vi "PromVIEW_GlobalInit.vi"(11 "Item Ref":T1) -> ()   [LabVIEW 2020]
uses:
  <resource>/Framework/Providers/API/ItemRef.ctl
  <resource>/Framework/Providers/API/mxLvMenuItem.ctl
panel:
  out "error out":errorcluster
  in  "error in":errorcluster
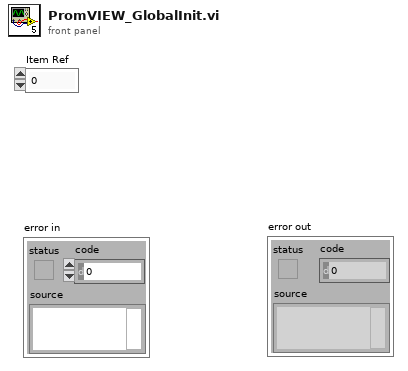
[diagram p1: front panel]
types:
  T1 = typedef "ItemRef.ctl" = u64
  T2 = enum32{"<None>", "Project", "Project / Build Specifications", "Tools", "Tools / Source Control", "Tools / Real-Time Module", "Help"}
  T3 = typedef "mxLvMenuItem.ctl" = cluster{"Menu Name":string, "Description":string, "Icon File Name":path, "Menu Tag":string, "Enabled":bool, "Checked":bool, "Separator":bool, "Batchable":bool, "Weight":i32, "Batch Mode (Ignored if Not Batchable)":enum32{"Show If All Items Support Command", "Show If Any Items Support Command"}, "Menu Location":enum32{"<None>", "Project", "Project / Build Specifications", "Tools", "Tools / Source Control", "Tools / Real-Time Module", "Help"}, "Exclude From Getting Started Window Menu":bool}
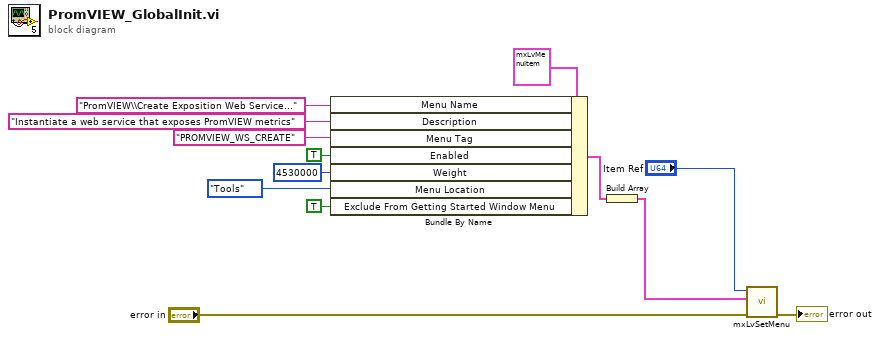
[diagram p0: block diagram]
diagram:
  n1 = Bundle By Name(cluster=T3 {"Menu Name"="", "Description"="", "Icon File Name"=path "", "Menu Tag"="", "Enabled"=TRUE, "Checked"=FALSE, "Separator"=FALSE, "Batchable"=TRUE, "Weight"=0, "Batch Mode (Ignored if Not Batchable)"=enum."Show If All Items Support Command", "Menu Location"=enum."<None>", "Exclude From Getting Started Window Menu"=FALSE} ("Menu Item"), "Menu Name"="PromVIEW\\Create Exposition Web Service...", "Description"="Instantiate a web service that exposes PromVIEW metrics", "Menu Tag"="PROMVIEW_WS_CREATE", "Enabled"=TRUE, "Weight"=4530000, "Menu Location"=T2."Tools", "Exclude From Getting Started Window Menu"=TRUE) -> (w9:T3)
  n2 = Build Array(w9) -> (w1:T3[])
  n3 = call <resource>:"mxLvSetMenu.vi"("error in"="error in", "Menu Items"=w1, "Item"="Item Ref") -> ("error out"=→"error out":errorcluster)  [unwired: 7 in, 1 out]
